vi "example 4 - string.vi"() -> ()   [LabVIEW 2020]
uses:
  ui-testing/ui-testing.lvlib
panel:
  in  "Tree":string[](tree)
  in  "String":string
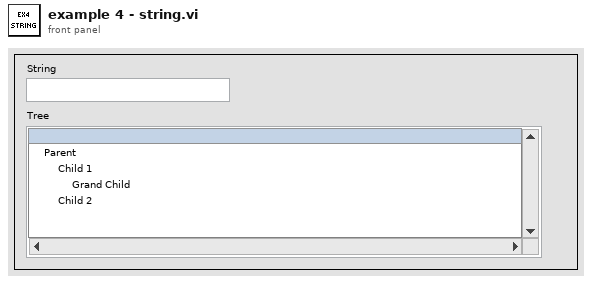
[diagram p1: front panel]
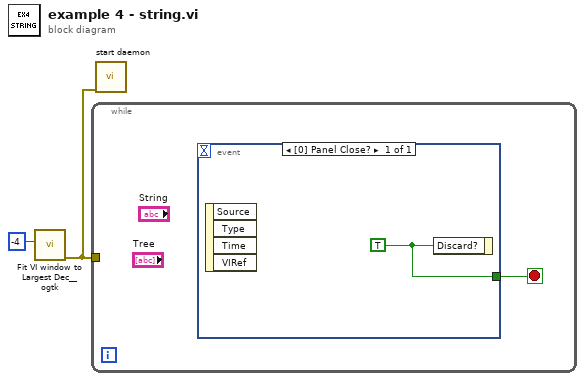
[diagram p0: block diagram]
diagram:
  n1 = call <userlib>:"Fit VI window to Largest Dec__ogtk.vi"("border spacing (2 px)"=-4) -> ("error out"=w1:errorcluster)  [unwired: 5 in, 1 out]
  n2 = while {
    tunnel: w1 -> [_]
    stop <- w3 stop-if-true
    n3 = event shown="[0] Panel Close?" {
      selector: _ -> [_]
      dyn-events: _ -> [_]
      timeout: _ -> [_]
      tunnel: [w4] -> w3
      event Panel Close? {
        w4 = TRUE
        n4 = event-data() -> ()  [unwired: 1 in, 4 out]
        n5 = event-data("Discard?"=w4) -> ()  [unwired: 1 in, 1 out]
      }
    }
  }
  n6 = call "start daemon.vi"("error in (no error)"=w1) -> ()  [unwired: 10 in, 1 out]
